vi "ListaTematy.vi"(7 "Jsonconfig":string, 8 "error in (no error)":errorcluster) -> (0 "error out":errorcluster, 2 "data":string[][](array[string]), 3 "Array":string[](array[string]))   [LabVIEW 2015]
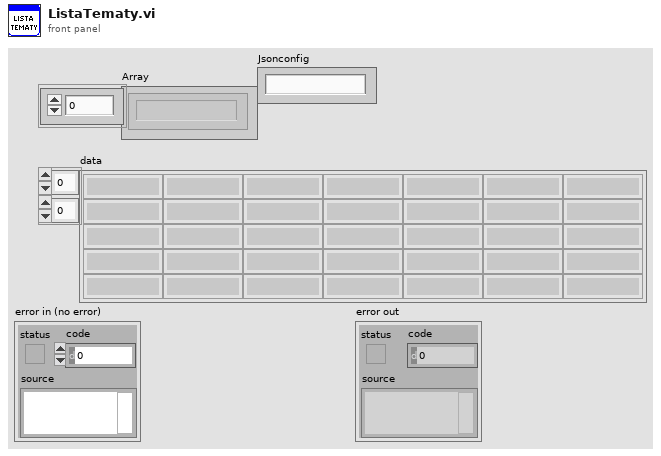
[diagram p1: front panel]
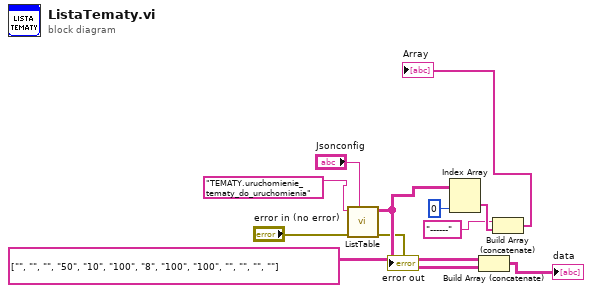
[diagram p0: block diagram]
diagram:
  n1 = call "ListTable.vi"("Jsonconfig"="Jsonconfig", "error in (no error)"="error in (no error)", "table"="TEMATY.uruchomienie_tematy_do_uruchomienia") -> ("error out"=→"error out":errorcluster, "data"=w3:string[][])  [unwired: 7 in]
  n2 = Index Array(array=w3, index (col)=0 ("disabled index (col)")) -> (element=w10:string[])  [unwired: 1 in]
  n3 = Build Array (concatenate)(string[][] [["", "", "", "50", "10", "100", "8", "100", "100", "", "", "", ""]] ("data"), w3) -> (→"data":string[][])
  n4 = Build Array (concatenate)("------", w10) -> (→"Array":string[])
